vi "ADC INL_sweep_working.vi"(8 "error in (no error)":errorcluster, 9 "Sequence parameters":string[][](array[string])=[["Min limit", "Max limit", "Register sheet file", "Register Sheet"], ["", "", "CC2600.xls", "TX_BLE;Trim"], ["Reg write (addr;value)", "Operating frequency [Hz]", "", ""], ["NA", "2.44G", "", ""]], 10 "Run type":i32, 11 "Method parameters":T4={"Dev"={"Do not disturb DUT"=FALSE, "XOSC"=32000000.0, "Board type"="", "EM"="", "Configure tempboard"=TRUE, "Device specific info"=[], "Generic Object"=refnum}, "Method"={"Run type"=1, "Test name"="Current LPM2 4", "Comment"="", "Results folder"="", "AFC"=enum."Off", "Method name"="Current LPM2 4", "Method results"={"Excel brief report"=FALSE, "Spotfire report"=FALSE, "Starfish report"=FALSE}, "Operator"="", "Reference time"=timestamp(0 s since 1904-01-01), "AFC delay"=0.0, "Initialization"=enum."Enabled", "MD5 Sum"="", "HW addon board"=enum."None", "AFC Regsheet"="", "AFC Regfile"=path "", "dummy"=0.0}, "Inst"={"Instr"={"PS1"={"Name"="", "GPIB address"="", "VISA session"=""}, "PS2"={"Name"="", "GPIB address"="", "VISA session"=""}, "TC1"={"Name"="", "GPIB address"="", "VISA session"=""}, "TC2"={"Name"="", "GPIB address"="", "VISA session"=""}, "SA1"={"Name"="", "GPIB address"="", "VISA session"=""}, "SA2"={"Name"="", "GPIB address"="", "VISA session"=""}, "SG1"={"Name"="", "GPIB address"="", "VISA session"=""}, "SG2"={"Name"="", "GPIB address"="", "VISA session"=""}, "SG3"={"Name"="", "GPIB address"="", "VISA session"=""}, "MI1"={"Name"="", "GPIB address"="", "VISA session"=""}, "MI2"={"Name"="", "GPIB address"="", "VISA session"=""}, "SW SA"={"Name"="", "Controller addr"=""}, "SW SG"={"Name"="", "Controller addr"=""}, "MI3"={"Name"="", "GPIB address"="", "VISA session"=""}}, "Switchbox"={"RF Path"=0, "Cal compensation"=enum."TX", "Switchbox gain mode"="", "State"=enum."TX"}, "Instr to control (i.e. SA1)"="Default", "Intrument info string"=""}, "Sequence parameters"=[["Weight", "Min Limit", "Max Limit", "Register Sheet", "", "", "", "", "", "", "", "", ""], ["Vital", "", "1", "LPM2", "", "", "", "", "", "", "", "", ""], ["Resolution", "Reg write (addr;value)", "Chip mode", "Range", "", "", "", "", "", "", "", "", ""], ["u", "NA", "", "auto", "", "", "", "", "", "", "", "", ""]], "Cond"={"Temp logged"=25.0, "VDD1_PS1_6V"=-999.0, "VDD2_PS1_25V"=-999.0, "VDD4_PS2_25V"=-999.0, "VDD3_PS2_6V"=-999.0}, "Meas config"={"X-axis inner loop index"=32000000, "Y-axis outer loop index"=32000000, "X-axis"=[], "Y-axis"=[], "X-axis array req size"=32000000, "Y-axis array req size"=32000000, "Param description"=[], "Use meas clust for reporting"=FALSE, "Parameter index (page)"=0, "X-axis name"="", "Y-axis name"=""}} {"Cond"."VDD3_PS2_6V" format="%.3f"; "Cond"."VDD4_PS2_25V" format="%.3f"; "Cond"."VDD2_PS1_25V" format="%.3f"; "Cond"."VDD1_PS1_6V" format="%.3f"; "Method"."dummy" format="%.1p"; "Method"."AFC delay" format="%.1p"; "Dev"."XOSC" format="%.3p"}) -> (0 "error out":errorcluster, 1 "End method error":T3, 2 "Short Results":string[](array[string])=["0.00", "0.00", "0.00", "0.00"], 3 "Result summary":string[][](array[string])=[["Critical", "Output Power@2405 MHz", "-3", "4", "dBm"], ["Critical", "Output Power@2410 MHz", "-3", "4", "dBm"]])   [LabVIEW 2019]
doc: "[AutoDocStart]Performs crystal accuracy measurements. Measures the offset from ideal frequency. Primarily used for tuning XOSC capacitors and verifying XOSC trims.\n\nSweeping parameters: operating frequency, OSC override value and VDDR level\n\nResults: Offset frequency in ppm[AutoDocEnd]"
uses:
  User Lib/Utilities/Cluster definitions/Method input.ctl
  User Lib/Utilities/Cluster definitions/Device specific info.ctl
  User Lib/Utilities/Controls/Automatic Frequency Compensation types.ctl
  User Lib/Utilities/Controls/Method Reports.ctl
  User Lib/Utilities/Cluster definitions/Method Initialization.ctl
  User Lib/Utilities/Controls/HW addon boards.ctl
  User Lib/Utilities/Cluster definitions/Instr clust.ctl
  User Lib/Utilities/Switchbox control/SwitchBox_State._ENUMctl.ctl
  User Lib/Utilities/Cluster definitions/End method error cluster.ctl
  User Lib/Utilities/Cluster definitions/DUT vdd control.ctl
  User Lib/Utilities/Cluster definitions/DUT VDD4.ctl
  User Lib/Utilities/Cluster definitions/DUT VDD3.ctl
  User Lib/Utilities/Cluster definitions/DUT VDD2.ctl
  User Lib/Utilities/Cluster definitions/DUT VDD1.ctl
  955d3981-8086-4abc-a4a1-ffeabbc67de4.vi
  ad5dbd7b-cdfb-4125-adc4-1165e2874c87.vi
  dbdc58e7-b514-4632-b463-1ba2de0afab7.vi
  5201a9fb-abbc-4d1d-b83d-08253667edc6.vi
panel:
  out "output cluster 8":T1={"Average Hits \nper Code "=198.76479217603912, "Min DNL"=-0.30764433555407467, "Min INL"=-0.5231398172109945, "Max INL"=0.7801825995135989, "Max DNL"=0.8022935268616486, "DNL Range"=0.5549689312078616, "INL Range"=0.6516612083622967}
  out "ADC samples 8":u32[](array[numeric])
  out "output cluster 7":T1={"Average Hits \nper Code "=198.76479217603912, "Min DNL"=-0.30764433555407467, "Min INL"=-0.5231398172109945, "Max INL"=0.7801825995135989, "Max DNL"=0.8022935268616486, "DNL Range"=0.5549689312078616, "INL Range"=0.6516612083622967}
  out "ADC samples 7":u32[](array[numeric])
  out "output cluster 5":T1={"Average Hits \nper Code "=198.76479217603912, "Min DNL"=-0.30764433555407467, "Min INL"=-0.5231398172109945, "Max INL"=0.7801825995135989, "Max DNL"=0.8022935268616486, "DNL Range"=0.5549689312078616, "INL Range"=0.6516612083622967}
  out "ADC samples 5":u32[](array[numeric])
  out "output cluster 4":T1={"Average Hits \nper Code "=198.76479217603912, "Min DNL"=-0.30764433555407467, "Min INL"=-0.5231398172109945, "Max INL"=0.7801825995135989, "Max DNL"=0.8022935268616486, "DNL Range"=0.5549689312078616, "INL Range"=0.6516612083622967}
  out "ADC samples 4":u32[](array[numeric])
  in  "Tab Control":T2(tab)
  # "°C"
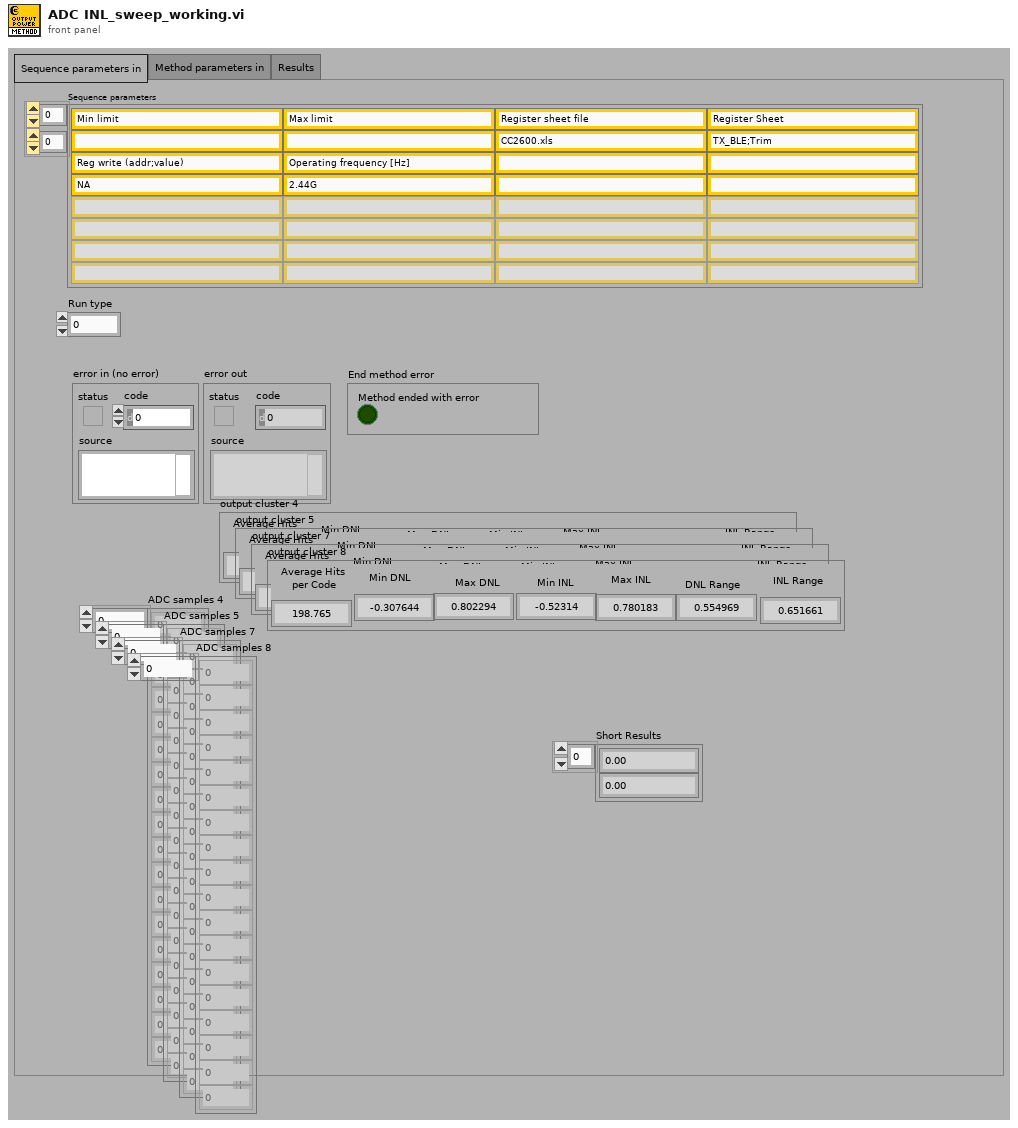
[diagram p1: front panel]
types:
  T1 = cluster{"Average Hits \nper Code ":dbl, "Min DNL":dbl, "Min INL":dbl, "Max INL":dbl, "Max DNL":dbl, "DNL Range":dbl, "INL Range":dbl}
  T2 = enum32{"Sequence parameters in", "Method parameters in", "Results"}
  T3 = typedef "End method error cluster.ctl" = cluster{"Method ended with error":bool}
  T4 = typedef "Method input.ctl" = cluster{"Dev":cluster{"Do not disturb DUT":bool, "XOSC":dbl, "Board type":string, "EM":string, "Configure tempboard":bool, "Device specific info":T5[], "Generic Object":refnum<class>}, "Method":cluster{"Run type":i32, "Test name":string, "Comment":string, "Results folder":string, "AFC":T6, "Method name":string, "Method results":T7, "Operator":string, "Reference time":timestamp, "AFC delay":dbl, "Initialization":T8, "MD5 Sum":string, "HW addon board":T9, "AFC Regsheet":string, "AFC Regfile":path, "dummy":dbl}, "Inst":T10, "Sequence parameters":string[][], "Cond":cluster{"Temp logged":dbl, "VDD1_PS1_6V":dbl, "VDD2_PS1_25V":dbl, "VDD4_PS2_25V":dbl, "VDD3_PS2_6V":dbl}, "Meas config":cluster{"X-axis inner loop index":i32, "Y-axis outer loop index":i32, "X-axis":string[], "Y-axis":string[], "X-axis array req size":i32, "Y-axis array req size":i32, "Param description":string[][], "Use meas clust for reporting":bool, "Parameter index (page)":i32, "X-axis name":string, "Y-axis name":string}}
  T5 = typedef "Device specific info.ctl" = cluster{"EM number":u8, "IP address":string, "Enabled":bool, "Slot no":u8, "RF path":u8, "EM name":string, "Wafer info":string, "AFC frequency ppm":dbl, "Register writes":string[][], "Meas data":string[][][], "Device comment":string}
  T6 = typedef "Automatic Frequency Compensation types.ctl" = enum16{"Off", "Compensate Instrument frequency", "Compensate DUT frequency", "Predictive - Compensate Instrument frequency", "Predictive - Compensate DUT frequency", "Do not skip re-init - Compensate Instrument frequency", "Do not skip re-init - Compensate DUT frequency"}
  T7 = typedef "Method Reports.ctl" = cluster{"Excel brief report":bool, "Spotfire report":bool, "Starfish report":bool}
  T8 = typedef "Method Initialization.ctl" = enum16{"Enabled", "Skip Instr and Device Init", "Enabled with Separate Flash", "Set PS, Device Init and Skip Instr Init", "Skip Device Init"}
  T9 = typedef "HW addon boards.ctl" = enum16{"None", "Current meas 5EM", "Stresstest 10EM"}
  T10 = typedef "Instr clust.ctl" = cluster{"Instr":cluster{"PS1":cluster{"Name":string, "GPIB address":string, "VISA session":refnum<visa-resource-name>}, "PS2":cluster{"Name":string, "GPIB address":string, "VISA session":refnum<visa-resource-name>}, "TC1":cluster{"Name":string, "GPIB address":string, "VISA session":refnum<visa-resource-name>}, "TC2":cluster{"Name":string, "GPIB address":string, "VISA session":refnum<visa-resource-name>}, "SA1":cluster{"Name":string, "GPIB address":string, "VISA session":refnum<visa-resource-name>}, "SA2":cluster{"Name":string, "GPIB address":string, "VISA session":refnum<visa-resource-name>}, "SG1":cluster{"Name":string, "GPIB address":string, "VISA session":refnum<visa-resource-name>}, "SG2":cluster{"Name":string, "GPIB address":string, "VISA session":refnum<visa-resource-name>}, "SG3":cluster{"Name":string, "GPIB address":string, "VISA session":refnum<visa-resource-name>}, "MI1":cluster{"Name":string, "GPIB address":string, "VISA session":refnum<visa-resource-name>}, "MI2":cluster{"Name":string, "GPIB address":string, "VISA session":refnum<visa-resource-name>}, "SW SA":cluster{"Name":string, "Controller addr":string}, "SW SG":cluster{"Name":string, "Controller addr":string}, "MI3":cluster{"Name":string, "GPIB address":string, "VISA session":refnum<visa-resource-name>}}, "Switchbox":cluster{"RF Path":i32, "Cal compensation":enum16{"TX", "RX", "Interferer", "No compensation", "Interferer2"}, "Switchbox gain mode":string, "State":T11}, "Instr to control (i.e. SA1)":string, "Intrument info string":string}
  T11 = typedef "SwitchBox_State._ENUMctl.ctl" = enum16{"TX", "RX", "SP:TX", "SP:RX", "SW:TX", "SW:RX"}
  T12 = typedef "DUT vdd control.ctl" = cluster{"VDD4 config":T13, "VDD3 config":T14, "VDD2 config":T15, "VDD1 config":T16}
  T13 = typedef "DUT VDD4.ctl" = u16
  T14 = typedef "DUT VDD3.ctl" = u16
  T15 = typedef "DUT VDD2.ctl" = u16
  T16 = typedef "DUT VDD1.ctl" = u16
  T17 = enum32{"NI Card Settings", "Memory Read Setting", "DC Capture", "ADC Ramp", "ADC Sine", "SNR", "Cap Calibration"}
  T18 = enum32{"Read from Memory", "Read .dat file", "NI Card Capture", "None"}
  T19 = cluster{"Path to Save plot":path, "Path to Raw Data plot":path}
  T20 = cluster{"Save INL/DNL Plot(Ramp)":bool, "Save SNR Plot":bool, "Save INL/DNL Plot(Sine)":bool, "Save INL/DNL Raw Data(Ramp)":bool, "Save SNR Raw Data":bool, "Save INL/DNL Raw Data(Sine)":bool, "Save DC Raw data":bool, "Save  Raw Data(Sine)":bool}
  T21 = cluster{"Min INL":dbl, "Max INL":dbl, "Min DNL":dbl, "Max DNL":dbl, "INL Range":dbl, "DNL Range":dbl, "Avg Hits/Code":dbl}
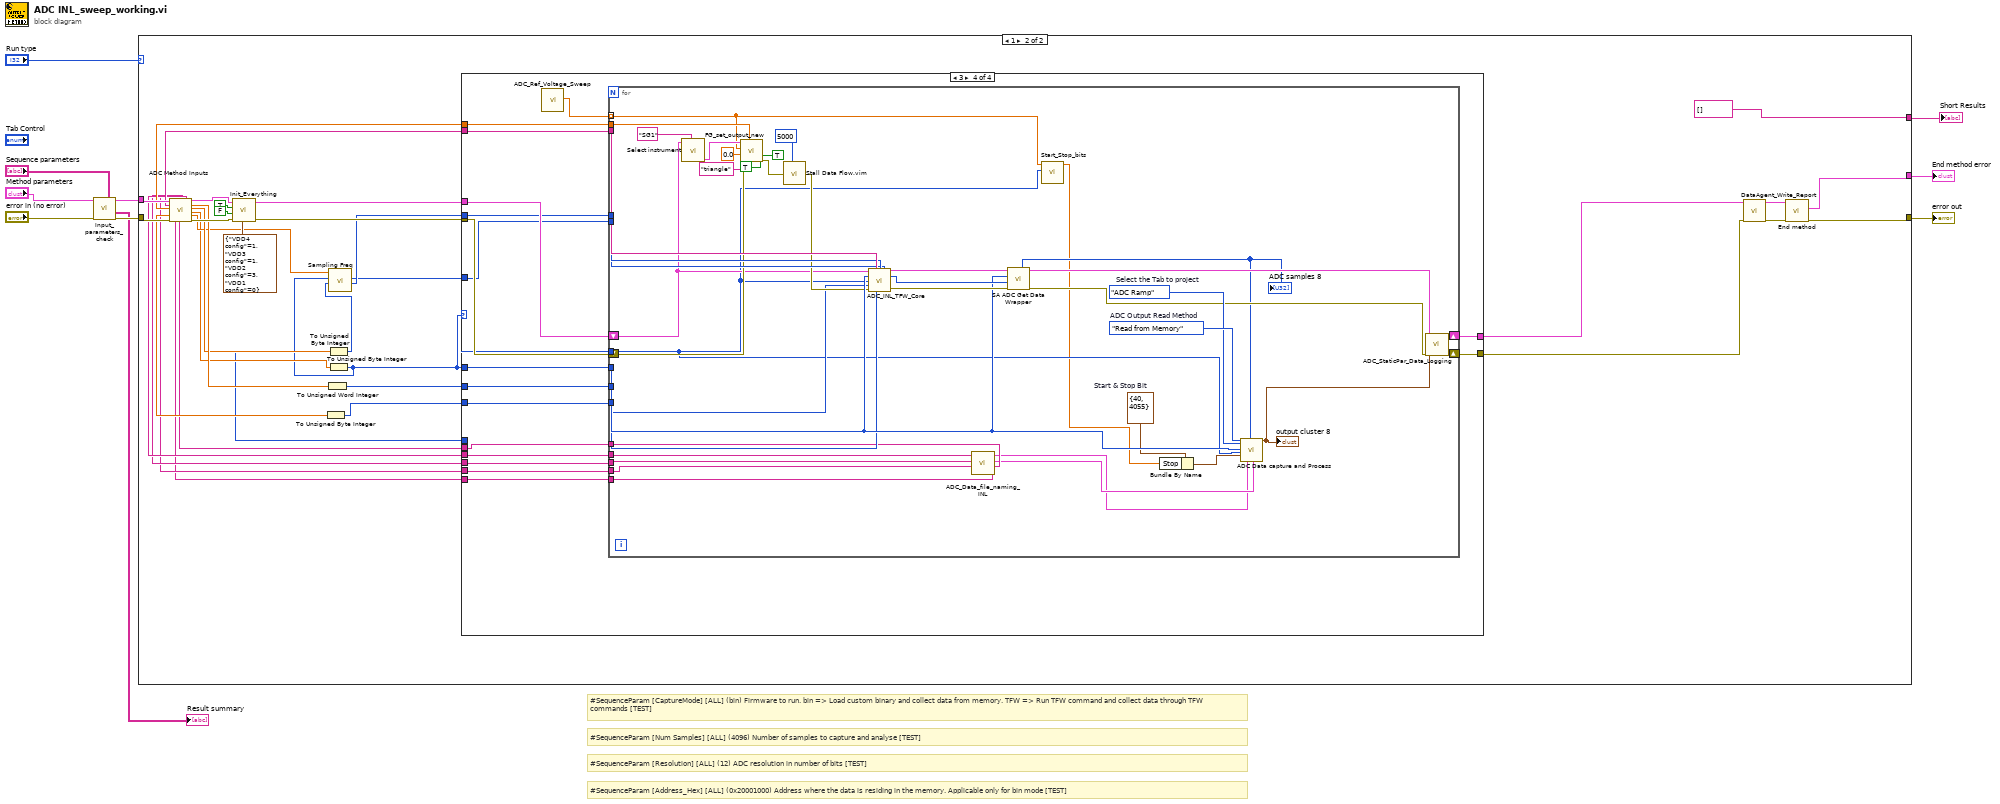
[diagram p0: block diagram]
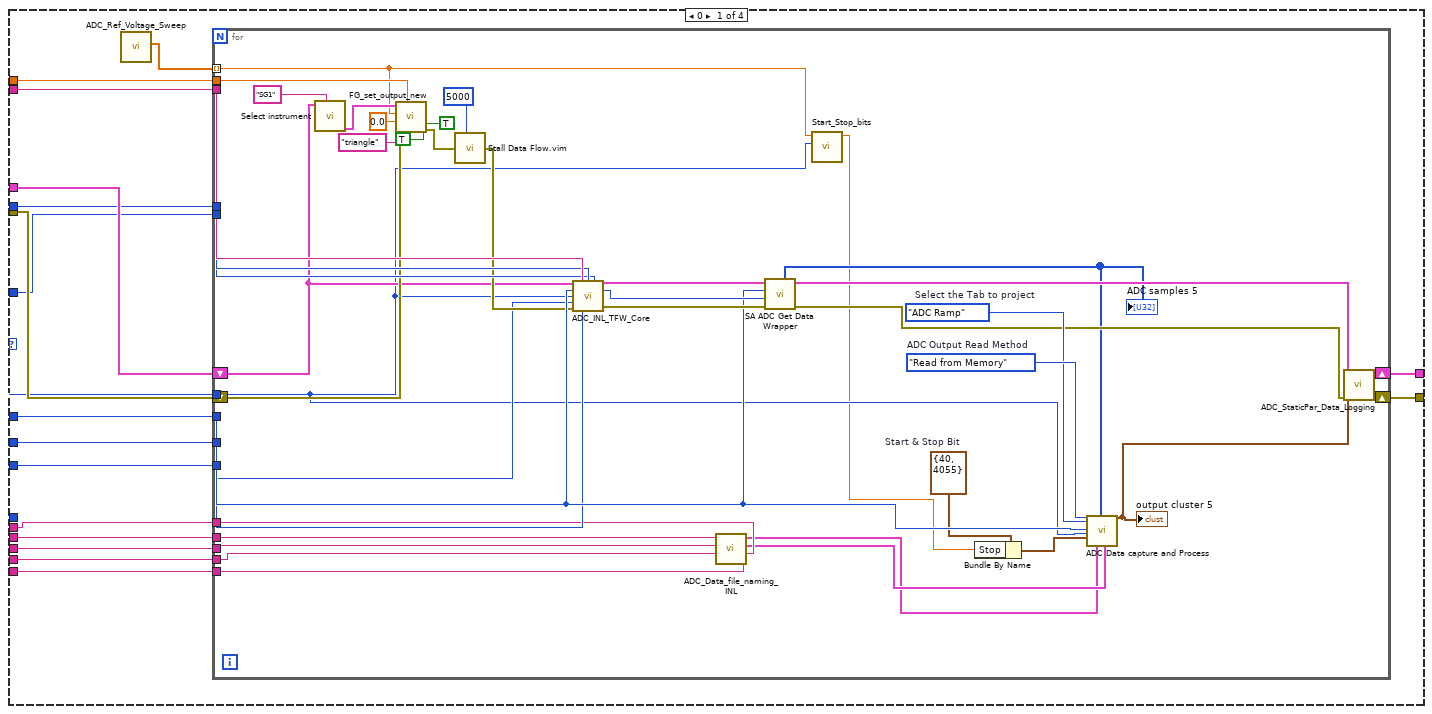
[diagram p3: hidden frame]
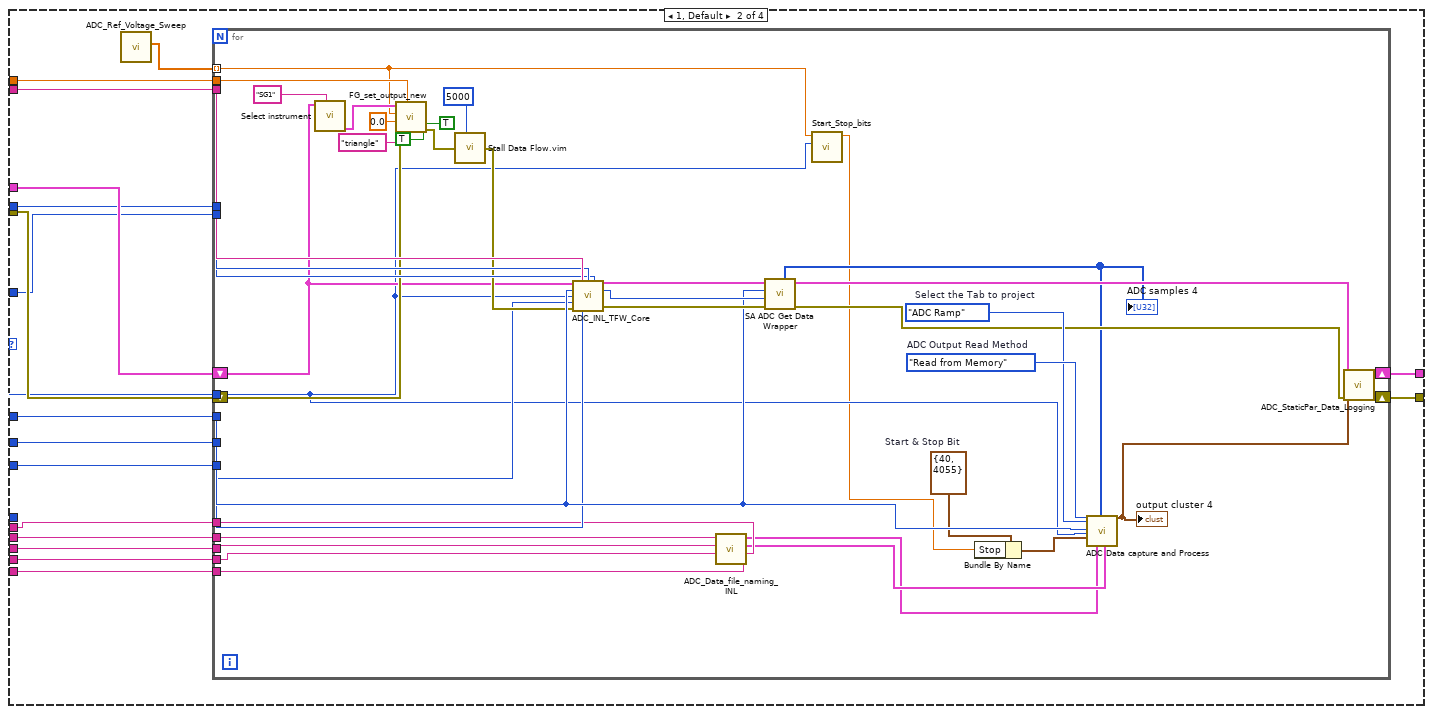
[diagram p4: hidden frame]
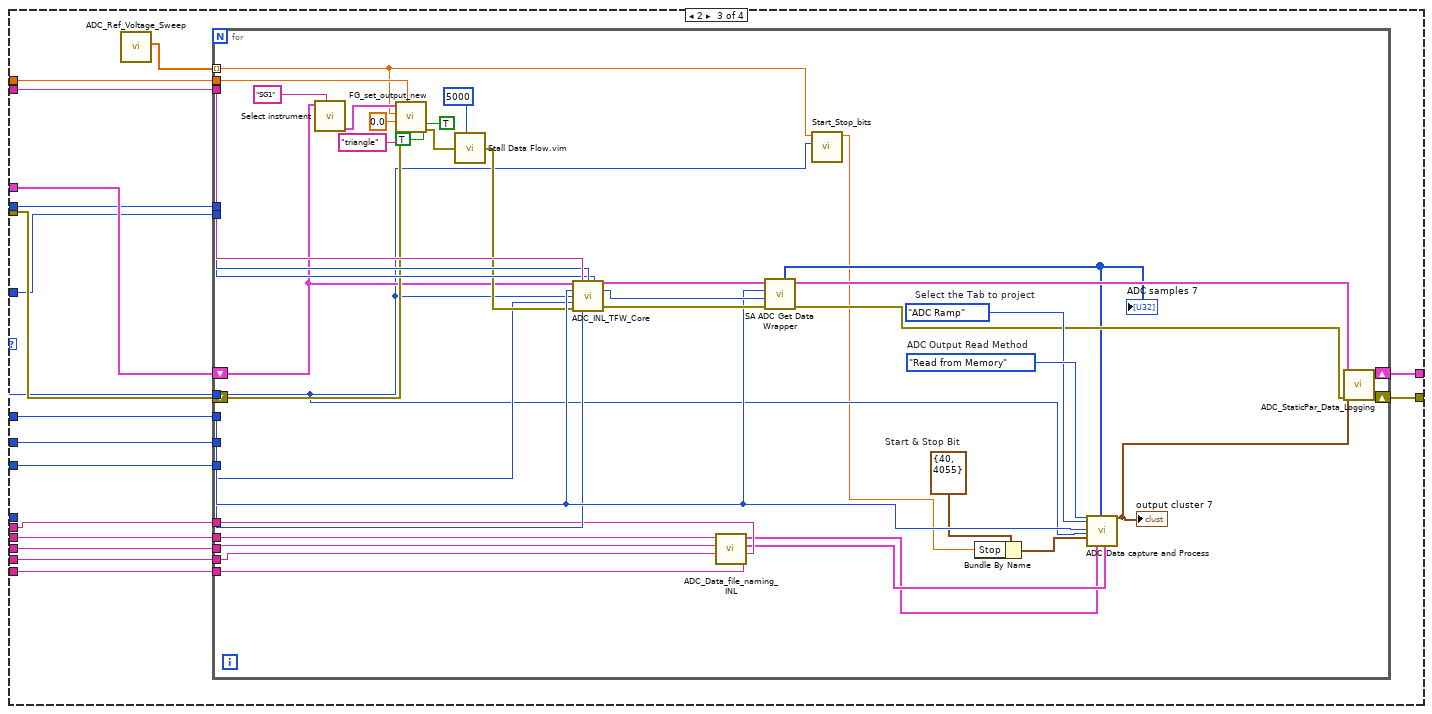
[diagram p5: hidden frame]
diagram:
  # "#SequenceParam [Num Samples] [ALL] (4096) Number of samples to capture and analyse [TEST]"
  # "#SequenceParam [CaptureMode] [ALL] (bin) Firmware to run. bin => Load custom binary and collect data from memory. TFW => Run TFW command and collect data through TFW commands [TEST]"
  # "#SequenceParam [Address_Hex] [ALL] (0x20001000) Address where the data is residing in the memory. Applicable only for bin mode [TEST]"
  # "#SequenceParam [Resolution] [ALL] (12) ADC resolution in number of bits [TEST]"
  n1 = call "Input_parameters_check.vi"("Sequence parameters"="Sequence parameters", "error in"="error in (no error)", "Method cluster in"="Method parameters") -> ("error out"=w9:errorcluster, "Result summary"=→"Result summary":string[][], "Method cluster out"=w5:T4)  [unwired: 6 in]
  n2 = case shown="1" "Run type" {
    tunnel: w9 -> [w11 w34]
    tunnel: [w11 w45] -> w10
    tunnel: w5 -> [_ w35]
    tunnel: [_ w44] -> w4
    tunnel: [_ string[] []] -> w1
    frame 0, Default {
      # "Run type 0 is only for formatting the result summary"
    }
    frame 1 {
      n3 = call "ADC Method Inputs.vi"("Method cluster in"=w35, "error in (no error)"=w34) -> ("Capture Mode"=w21:string, "Signal Freq"=w17:dbl, "ADC Chnl No."=w27:dbl, "Input Voltage String"=w13:string, "Sampling Freq String"=w14:string, "Chnl No. string"=w12:string, "Resolution String"=w15:string, "Voltage Ref String"=w16:string, "Method cluster out"=w32:T4, "Num Samples"=w31:dbl, "Resolution"=w30:dbl, "Voltage Ref"=w28:dbl, "Sampling Freq"=w29:dbl, "error out"=w33:errorcluster)  [unwired: 2 in, 2 out]
      n4 = call "Init_Everything.vi"("VDD config"=T12 {"VDD4 config"=1, "VDD3 config"=1, "VDD2 config"=3, "VDD1 config"=0}, "error in"=w33, "Support current measurement?"=FALSE, "Override VDD Config"=TRUE, "Method cluster In"=w32) -> ("error out"=w25:errorcluster, "Method cluster out"=w26:T4)  [unwired: 3 in, 2 out]
      n5 = To Unsigned Byte Integer(number=w27) -> (unsigned 8bit integer=w22:u8)
      n6 = To Unsigned Word Integer(number=w31) -> (unsigned 16bit integer=w24:u16)
      n7 = To Unsigned Byte Integer(number=w30) -> (unsigned 8bit integer=w23:u8)
      n8 = To Unsigned Byte Integer(number=w28) -> (unsigned 8bit integer=w18:u8)
      n9 = call "Sampling Freq.vi"("Resolution"=w23, "Voltage Ref"=w18, "Sampling Freq"=w29) -> ("LGPT Count"=w20:u16, "SCOMP"=w19:u16)  [unwired: 7 in]
      n10 = case shown="3" w18 {
        tunnel: [w63 w122 w181 w240] -> w39
        tunnel: [w62 w121 w180 w239] -> w38
        tunnel: w26 -> [w61 w120 w179 w238]
        tunnel: w25 -> [w60 w119 w178 w237]
        tunnel: w24 -> [w59 w118 w177 w236]
        tunnel: w23 -> [w58 w117 w176 w235]
        tunnel: w18 -> [w57 w116 w175 w234]
        tunnel: w22 -> [w56 w115 w174 w233]
        tunnel: w21 -> [w55 w114 w173 w232]
        tunnel: w20 -> [w54 w113 w172 w231]
        tunnel: w19 -> [w53 w112 w171 w230]
        tunnel: w17 -> [w51 w110 w169 w228]
        tunnel: w16 -> [w50 w109 w168 w227]
        tunnel: w15 -> [w49 w108 w167 w226]
        tunnel: w14 -> [w48 w107 w166 w225]
        tunnel: w13 -> [w47 w106 w165 w224]
        tunnel: w12 -> [w46 w105 w164 w223]
        frame 0 {
          n11 = call "ADC_Ref_Voltage_Sweep.vi"() -> ("Ref voltage sweep"=w52:dbl[])  [unwired: 11 in]
          n12 = for {
            tunnel: w59 -> [w93]
            tunnel: w58 -> [w68]
            tunnel: w57 -> [w69]
            tunnel: w56 -> [w92]
            tunnel: w55 -> [w91]
            tunnel: w54 -> [w90]
            tunnel: w53 -> [w89]
            shift-right: [w99] -> w63
            shift-left: w61 -> [w83]
            shift-right: [w98] -> w62
            shift-left: w60 -> [w86]
            tunnel: w52 -> [w67] mode=indexing
            tunnel: w51 -> [w79]
            tunnel: w50 -> [w76]
            tunnel: w49 -> [w75]
            tunnel: w48 -> [w74]
            tunnel: w47 -> [w73]
            tunnel: w46 -> [w72]
            w66 = cluster{"Start":i32, "Stop":i32} {"Start"=40, "Stop"=4055}  # Start & Stop Bit
            w103 = T17."ADC Ramp"  # Select the Tab to project
            w104 = T18."Read from Memory"  # ADC Output Read Method
            n13 = call "Select instrument.vi"("Instr.Instr to control (i.e. SA1)"="SG1", "Method cluster in"=w83) -> ("Instr out"=w88:T10)  [unwired: 7 in, 2 out]
            n14 = call "FG_set_output_new.vi"("High impedance (T)"=TRUE, "Enable Output?"=TRUE, "Function (DC, Sine, Square, Triangle, Ramp up, Ramp down, Pulse)"="triangle", "Frequency [Hz]"=w79, "error in"=w86, "Low voltage"=0.0, "High voltage (or DC)"=w67, "InstrCluster in"=w88) -> ("error out"=w85:errorcluster)  [unwired: 2 in, 1 out]
            n15 = call "Stall Data Flow.vim"("value in"=w85, "milliseconds to wait"=u32 5000) -> ("value out"=w84:errorcluster)  [unwired: 1 out]
            n16 = call "ADC_INL_TFW_Core.vi"("Method cluster in"=w83, "Capture Mode"=w91, "LGPT Count"=w90, "SCOMP"=w89, "No. Samples"=w93, "Resolution"=w68, "Voltage Ref"=w69, "error in"=w84, "ADC Chnl No."=w92) -> ("Method cluster out"=w95:T4, "ResPar[0] Data Address"=w94:u32, "error out"=w96:errorcluster)  [unwired: 3 in, 1 out]
            n17 = call "ADC_Data_file_naming_INL.vi"("Amplitude (Vpp)"=w73, "ADC Chn. No"=w72, "Sampling Freq String"=w74, "Resolution String"=w75, "Voltage Ref String"=w76) -> ("path to save"=w71:T19, "Save data"=w70:T20)  [unwired: 5 in]
            n18 = call "SA ADC Get Data Wrapper.vi"("error in"=w96, "Data Address"=w94, "Num Samples"=w93, "Method cluster in"=w95) -> ("error out"=w102:errorcluster, "output cluster"=w101:T4, "ADC samples"=w100:u32[])  [unwired: 2 in, 3 out]
            "ADC samples 5" <- w100
            n19 = call "Start_Stop_bits.vi"("Resolution"=w68, "Input Amplitude"=w67) -> ("Stop Bit"=w64:dbl)  [unwired: 9 in]
            n20 = Bundle By Name(cluster=w66, "Stop"=w64) -> (w65:cluster{"Start":i32, "Stop":i32})
            n21 = call "ADC Data capture and Process.vi"("ADC Output Read Method"=w104, "Select the Tab to project"=w103, "No.of samples"=w93, "Resolution"=w68, "Start & Stop Bit"=w65, "Save data"=w70, "Input Waveform"=w100, "path to save"=w71) -> ("Static Parameters (Ramp)"=w97:T21)  [unwired: 14 in, 5 out]
            "output cluster 5" <- w97
            n22 = call "ADC_StaticPar_Data_Logging.vi"("error in (no error)"=w102, "Static Parameters (Ramp)"=w97, "output cluster"=w101) -> ("error out"=w98:errorcluster, "Method cluster out"=w99:T4)  [unwired: 7 in]
          }
        }
        frame 1, Default {
          n23 = call "ADC_Ref_Voltage_Sweep.vi"() -> ("Ref voltage sweep"=w111:dbl[])  [unwired: 11 in]
          n24 = for {
            tunnel: w118 -> [w152]
            tunnel: w117 -> [w127]
            tunnel: w116 -> [w128]
            tunnel: w115 -> [w151]
            tunnel: w114 -> [w150]
            tunnel: w113 -> [w149]
            tunnel: w112 -> [w148]
            shift-right: [w158] -> w122
            shift-left: w120 -> [w142]
            shift-right: [w157] -> w121
            shift-left: w119 -> [w145]
            tunnel: w111 -> [w126] mode=indexing
            tunnel: w110 -> [w138]
            tunnel: w109 -> [w135]
            tunnel: w108 -> [w134]
            tunnel: w107 -> [w133]
            tunnel: w106 -> [w132]
            tunnel: w105 -> [w131]
            w125 = cluster{"Start":i32, "Stop":i32} {"Start"=40, "Stop"=4055}  # Start & Stop Bit
            w162 = T17."ADC Ramp"  # Select the Tab to project
            w163 = T18."Read from Memory"  # ADC Output Read Method
            n25 = call "Select instrument.vi"("Instr.Instr to control (i.e. SA1)"="SG1", "Method cluster in"=w142) -> ("Instr out"=w147:T10)  [unwired: 7 in, 2 out]
            n26 = call "FG_set_output_new.vi"("High impedance (T)"=TRUE, "Enable Output?"=TRUE, "Function (DC, Sine, Square, Triangle, Ramp up, Ramp down, Pulse)"="triangle", "Frequency [Hz]"=w138, "error in"=w145, "Low voltage"=0.0, "High voltage (or DC)"=w126, "InstrCluster in"=w147) -> ("error out"=w144:errorcluster)  [unwired: 2 in, 1 out]
            n27 = call "Stall Data Flow.vim"("value in"=w144, "milliseconds to wait"=u32 5000) -> ("value out"=w143:errorcluster)  [unwired: 1 out]
            n28 = call "ADC_INL_TFW_Core.vi"("Method cluster in"=w142, "Capture Mode"=w150, "LGPT Count"=w149, "SCOMP"=w148, "No. Samples"=w152, "Resolution"=w127, "Voltage Ref"=w128, "error in"=w143, "ADC Chnl No."=w151) -> ("Method cluster out"=w154:T4, "ResPar[0] Data Address"=w153:u32, "error out"=w155:errorcluster)  [unwired: 3 in, 1 out]
            n29 = call "ADC_Data_file_naming_INL.vi"("Amplitude (Vpp)"=w132, "ADC Chn. No"=w131, "Sampling Freq String"=w133, "Resolution String"=w134, "Voltage Ref String"=w135) -> ("path to save"=w130:T19, "Save data"=w129:T20)  [unwired: 5 in]
            n30 = call "SA ADC Get Data Wrapper.vi"("error in"=w155, "Data Address"=w153, "Num Samples"=w152, "Method cluster in"=w154) -> ("error out"=w161:errorcluster, "output cluster"=w160:T4, "ADC samples"=w159:u32[])  [unwired: 2 in, 3 out]
            "ADC samples 4" <- w159
            n31 = call "Start_Stop_bits.vi"("Resolution"=w127, "Input Amplitude"=w126) -> ("Stop Bit"=w123:dbl)  [unwired: 9 in]
            n32 = Bundle By Name(cluster=w125, "Stop"=w123) -> (w124:cluster{"Start":i32, "Stop":i32})
            n33 = call "ADC Data capture and Process.vi"("ADC Output Read Method"=w163, "Select the Tab to project"=w162, "No.of samples"=w152, "Resolution"=w127, "Start & Stop Bit"=w124, "Save data"=w129, "Input Waveform"=w159, "path to save"=w130) -> ("Static Parameters (Ramp)"=w156:T21)  [unwired: 14 in, 5 out]
            "output cluster 4" <- w156
            n34 = call "ADC_StaticPar_Data_Logging.vi"("error in (no error)"=w161, "Static Parameters (Ramp)"=w156, "output cluster"=w160) -> ("error out"=w157:errorcluster, "Method cluster out"=w158:T4)  [unwired: 7 in]
          }
        }
        frame 2 {
          n35 = call "ADC_Ref_Voltage_Sweep.vi"() -> ("Ref voltage sweep"=w170:dbl[])  [unwired: 11 in]
          n36 = for {
            tunnel: w177 -> [w211]
            tunnel: w176 -> [w186]
            tunnel: w175 -> [w187]
            tunnel: w174 -> [w210]
            tunnel: w173 -> [w209]
            tunnel: w172 -> [w208]
            tunnel: w171 -> [w207]
            shift-right: [w217] -> w181
            shift-left: w179 -> [w201]
            shift-right: [w216] -> w180
            shift-left: w178 -> [w204]
            tunnel: w170 -> [w185] mode=indexing
            tunnel: w169 -> [w197]
            tunnel: w168 -> [w194]
            tunnel: w167 -> [w193]
            tunnel: w166 -> [w192]
            tunnel: w165 -> [w191]
            tunnel: w164 -> [w190]
            w184 = cluster{"Start":i32, "Stop":i32} {"Start"=40, "Stop"=4055}  # Start & Stop Bit
            w221 = T17."ADC Ramp"  # Select the Tab to project
            w222 = T18."Read from Memory"  # ADC Output Read Method
            n37 = call "Select instrument.vi"("Instr.Instr to control (i.e. SA1)"="SG1", "Method cluster in"=w201) -> ("Instr out"=w206:T10)  [unwired: 7 in, 2 out]
            n38 = call "FG_set_output_new.vi"("High impedance (T)"=TRUE, "Enable Output?"=TRUE, "Function (DC, Sine, Square, Triangle, Ramp up, Ramp down, Pulse)"="triangle", "Frequency [Hz]"=w197, "error in"=w204, "Low voltage"=0.0, "High voltage (or DC)"=w185, "InstrCluster in"=w206) -> ("error out"=w203:errorcluster)  [unwired: 2 in, 1 out]
            n39 = call "Stall Data Flow.vim"("value in"=w203, "milliseconds to wait"=u32 5000) -> ("value out"=w202:errorcluster)  [unwired: 1 out]
            n40 = call "ADC_INL_TFW_Core.vi"("Method cluster in"=w201, "Capture Mode"=w209, "LGPT Count"=w208, "SCOMP"=w207, "No. Samples"=w211, "Resolution"=w186, "Voltage Ref"=w187, "error in"=w202, "ADC Chnl No."=w210) -> ("Method cluster out"=w213:T4, "ResPar[0] Data Address"=w212:u32, "error out"=w214:errorcluster)  [unwired: 3 in, 1 out]
            n41 = call "ADC_Data_file_naming_INL.vi"("Amplitude (Vpp)"=w191, "ADC Chn. No"=w190, "Sampling Freq String"=w192, "Resolution String"=w193, "Voltage Ref String"=w194) -> ("path to save"=w189:T19, "Save data"=w188:T20)  [unwired: 5 in]
            n42 = call "SA ADC Get Data Wrapper.vi"("error in"=w214, "Data Address"=w212, "Num Samples"=w211, "Method cluster in"=w213) -> ("error out"=w220:errorcluster, "output cluster"=w219:T4, "ADC samples"=w218:u32[])  [unwired: 2 in, 3 out]
            "ADC samples 7" <- w218
            n43 = call "Start_Stop_bits.vi"("Resolution"=w186, "Input Amplitude"=w185) -> ("Stop Bit"=w182:dbl)  [unwired: 9 in]
            n44 = Bundle By Name(cluster=w184, "Stop"=w182) -> (w183:cluster{"Start":i32, "Stop":i32})
            n45 = call "ADC Data capture and Process.vi"("ADC Output Read Method"=w222, "Select the Tab to project"=w221, "No.of samples"=w211, "Resolution"=w186, "Start & Stop Bit"=w183, "Save data"=w188, "Input Waveform"=w218, "path to save"=w189) -> ("Static Parameters (Ramp)"=w215:T21)  [unwired: 14 in, 5 out]
            "output cluster 7" <- w215
            n46 = call "ADC_StaticPar_Data_Logging.vi"("error in (no error)"=w220, "Static Parameters (Ramp)"=w215, "output cluster"=w219) -> ("error out"=w216:errorcluster, "Method cluster out"=w217:T4)  [unwired: 7 in]
          }
        }
        frame 3 {
          n47 = call "ADC_Ref_Voltage_Sweep.vi"() -> ("Ref voltage sweep"=w229:dbl[])  [unwired: 11 in]
          n48 = for {
            tunnel: w236 -> [w270]
            tunnel: w235 -> [w245]
            tunnel: w234 -> [w246]
            tunnel: w233 -> [w269]
            tunnel: w232 -> [w268]
            tunnel: w231 -> [w267]
            tunnel: w230 -> [w266]
            shift-right: [w276] -> w240
            shift-left: w238 -> [w260]
            shift-right: [w275] -> w239
            shift-left: w237 -> [w263]
            tunnel: w229 -> [w244] mode=indexing
            tunnel: w228 -> [w256]
            tunnel: w227 -> [w253]
            tunnel: w226 -> [w252]
            tunnel: w225 -> [w251]
            tunnel: w224 -> [w250]
            tunnel: w223 -> [w249]
            w243 = cluster{"Start":i32, "Stop":i32} {"Start"=40, "Stop"=4055}  # Start & Stop Bit
            w280 = T17."ADC Ramp"  # Select the Tab to project
            w281 = T18."Read from Memory"  # ADC Output Read Method
            n49 = call "Select instrument.vi"("Instr.Instr to control (i.e. SA1)"="SG1", "Method cluster in"=w260) -> ("Instr out"=w265:T10)  [unwired: 7 in, 2 out]
            n50 = call "FG_set_output_new.vi"("High impedance (T)"=TRUE, "Enable Output?"=TRUE, "Function (DC, Sine, Square, Triangle, Ramp up, Ramp down, Pulse)"="triangle", "Frequency [Hz]"=w256, "error in"=w263, "Low voltage"=0.0, "High voltage (or DC)"=w244, "InstrCluster in"=w265) -> ("error out"=w262:errorcluster)  [unwired: 2 in, 1 out]
            n51 = call "Stall Data Flow.vim"("value in"=w262, "milliseconds to wait"=u32 5000) -> ("value out"=w261:errorcluster)  [unwired: 1 out]
            n52 = call "ADC_INL_TFW_Core.vi"("Method cluster in"=w260, "Capture Mode"=w268, "LGPT Count"=w267, "SCOMP"=w266, "No. Samples"=w270, "Resolution"=w245, "Voltage Ref"=w246, "error in"=w261, "ADC Chnl No."=w269) -> ("Method cluster out"=w272:T4, "ResPar[0] Data Address"=w271:u32, "error out"=w273:errorcluster)  [unwired: 3 in, 1 out]
            n53 = call "ADC_Data_file_naming_INL.vi"("Amplitude (Vpp)"=w250, "ADC Chn. No"=w249, "Sampling Freq String"=w251, "Resolution String"=w252, "Voltage Ref String"=w253) -> ("path to save"=w248:T19, "Save data"=w247:T20)  [unwired: 5 in]
            n54 = call "SA ADC Get Data Wrapper.vi"("error in"=w273, "Data Address"=w271, "Num Samples"=w270, "Method cluster in"=w272) -> ("error out"=w279:errorcluster, "output cluster"=w278:T4, "ADC samples"=w277:u32[])  [unwired: 2 in, 3 out]
            "ADC samples 8" <- w277
            n55 = call "Start_Stop_bits.vi"("Resolution"=w245, "Input Amplitude"=w244) -> ("Stop Bit"=w241:dbl)  [unwired: 9 in]
            n56 = Bundle By Name(cluster=w243, "Stop"=w241) -> (w242:cluster{"Start":i32, "Stop":i32})
            n57 = call "ADC Data capture and Process.vi"("ADC Output Read Method"=w281, "Select the Tab to project"=w280, "No.of samples"=w270, "Resolution"=w245, "Start & Stop Bit"=w242, "Save data"=w247, "Input Waveform"=w277, "path to save"=w248) -> ("Static Parameters (Ramp)"=w274:T21)  [unwired: 14 in, 5 out]
            "output cluster 8" <- w274
            n58 = call "ADC_StaticPar_Data_Logging.vi"("error in (no error)"=w279, "Static Parameters (Ramp)"=w274, "output cluster"=w278) -> ("error out"=w275:errorcluster, "Method cluster out"=w276:T4)  [unwired: 7 in]
          }
        }
      }
      n59 = call "DataAgent_Write_Report.vi"("error in (no error)"=w38, "Method cluster in"=w39) -> ("error out"=w42:errorcluster, "Method cluster out"=w41:T4)  [unwired: 8 in]
      n60 = call "End method.vi"("error in"=w42, "Method cluster in"=w41) -> ("error out"=w45:errorcluster, "End method error"=w44:T3)  [unwired: 7 in, 1 out]
    }
  }
  "error out" <- w10
  "End method error" <- w4
  "Short Results" <- w1
